vi "launchNewEditor.vi"(8 "error in (no error)":errorcluster, 10 "deviceDataBase":refnum<class "deviceDataBase.lvclass">, 11 "ScriptEditorV2 in":refnum<class "ScriptEditorV2.lvclass">) -> (0 "error out":errorcluster, 3 "ScriptEditorV2 out":refnum<class "ScriptEditorV2.lvclass">)   [LabVIEW 2011, in "Views.lvlib" / "ScriptEditor.lvlib" / "ScriptEditorV2.lvclass"]
uses:
  ScriptEditorV2.lvclass
  Tools/DatabaseHelpers/DbConnection/DeviceDataBase/deviceDataBase.lvclass
  ScriptEditorV2.lvclass/ScriptEditorV2.ctl
  Tools/Filing/FileSystem/FileSystem.lvclass
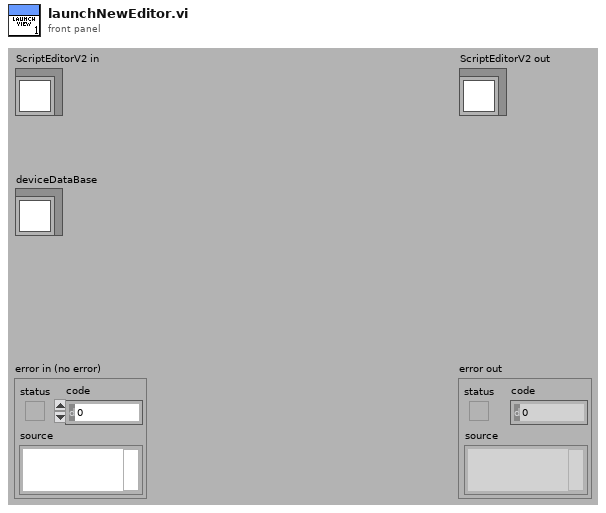
[diagram p1: front panel]
types:
  T1 = enum32{"Invalid", "Standard", "Closed", "Hidden", "Minimized", "Maximized"}
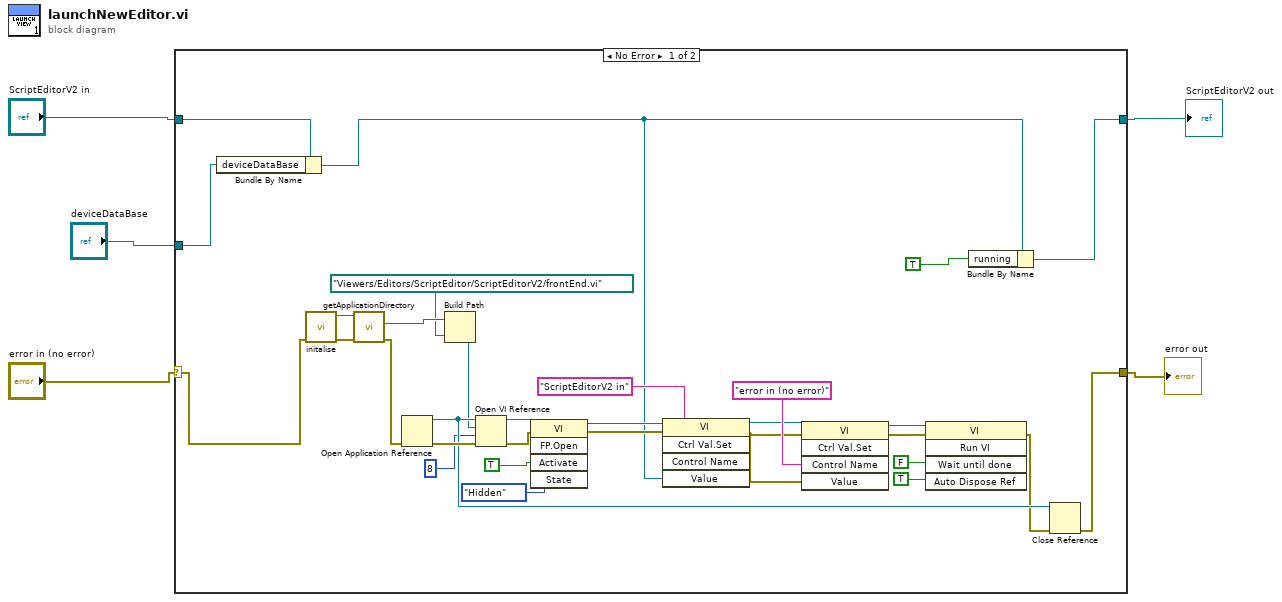
[diagram p0: block diagram]
diagram:
  n1 = case shown="No Error" "error in (no error)" {
    selector: "error in (no error)" -> [w9 w38]
    tunnel: [w28 w38] -> w2
    tunnel: "ScriptEditorV2 in" -> [w18 w37]
    tunnel: [w16 w37] -> w4
    tunnel: "deviceDataBase" -> [w19 _]
    frame No Error {
      n2 = Bundle By Name(cluster=w18, "deviceDataBase"=w19) -> (w14:refnum<class "ScriptEditorV2.lvclass">)
      n3 = call "initalise.vi"("error in (no error)"=w9) -> ("error out"=w11:errorcluster, "FileSystem out"=w10:refnum<class "FileSystem.lvclass">)  [unwired: 9 in]
      n4 = call-dynamic "getApplicationDirectory.vi"("error in (no error)"=w11, "FileSystem.lvclass in"=w10) -> ("error out"=w8:errorcluster, "ApplicationDirectory"=w13:path)  [unwired: 7 in, 1 out]
      n5 = Open Application Reference(8:w8) -> (0:w33:errorcluster, 3:w30:refnum<vi>)  [unwired: 3 in]
      n6 = Build Path(base path=w13, name or relative path=path "Viewers/Editors/ScriptEditor/ScriptEditorV2/frontEnd.vi" ("vi path")) -> (appended path=w7:path)
      n7 = Open VI Reference(application reference (local)=w30, vi path=w7, options=8, error in (no error)=w33) -> (vi reference=w25:refnum<vi>, error out=w24:errorcluster)  [unwired: 2 in]
      n8 = invoke class="VI" method="FP.Open"(reference=w25, error in=w24, "Activate"=TRUE, "State"=T1."Hidden") -> (reference out=w23:refnum<vi>, error out=w22:errorcluster)  [unwired: 1 in, 3 out]
      n9 = invoke class="VI" method="Ctrl Val.Set"(reference=w23, error in=w22, "Control Name"="ScriptEditorV2 in", "Value"=w14) -> (reference out=w32:refnum<vi>, error out=w31:errorcluster)  [unwired: 1 in, 3 out]
      n10 = invoke class="VI" method="Ctrl Val.Set"(reference=w32, error in=w31, "Control Name"="error in (no error)", "Value"=w31) -> (reference out=w27:refnum<vi>, error out=w26:errorcluster)  [unwired: 1 in, 3 out]
      n11 = invoke class="VI" method="Run VI"(reference=w27, error in=w26, "Wait until done"=FALSE, "Auto Dispose Ref"=TRUE) -> (error out=w29:errorcluster)  [unwired: 1 in, 4 out]
      n12 = Bundle By Name(cluster=w14, "running"=TRUE) -> (w16:refnum<class "ScriptEditorV2.lvclass">)
      n13 = Close Reference(reference=w30, error in (no error)=w29) -> (error out=w28:errorcluster)
    }
    frame Error {
    }
  }
  "error out" <- w2
  "ScriptEditorV2 out" <- w4
